vi "Teleop.vi"(10 "Match Info":T1={"Autonomous Elapsed Seconds"=0.0, "TeleOp Elapsed Seconds"=0.0, "Disabled Elapsed Seconds"=0.0, "Visited Autonomous"=FALSE, "Visited TeleOp"=FALSE, "Visited Disabled"=FALSE, "Autonomous Settings"={"Autonomous Style"=enum."Independent", "VI Refnum"=refnum}}, 11 "Call Context":T2) -> ()   [LabVIEW 2019]
doc: "This VI is called for each TeleOp packet received from the DS where the robot is not disabled. It is often used to read from the joysticks and update I/O or to update setpoints for timed control loops. It should complete and return within 20 milliseconds or it may miss DS packets."
uses:
  <vilib>/Rock Robotics/WPI/DriverStation/WPI_DriverStationDerivedRobotMode.ctl
  <vilib>/Rock Robotics/WPI/DriverStation/WPI_DriverStationMatch Info.ctl
  <vilib>/Rock Robotics/WPI/ThirdParty/Phoenix-LabVIEW/Motor Controller/Controls/CTRE_Phoenix_MotorControl_ControlMode.ctl
  <vilib>/Rock Robotics/WPI/Utilities/WPI_GetSetVariantRefNum.vi
  <vilib>/Rock Robotics/Network Tables/NT Write Boolean Array.vi
  <vilib>/Rock Robotics/Network Tables/NT Read Boolean.vi
  <vilib>/Rock Robotics/Network Tables/NT Read Number.vi
  <vilib>/Rock Robotics/Network Tables/NT Write Numeric Array.vi
panel:
  out "Sample Slider 0":dbl(slide) scale=0.0..5.0
  out "Sample Boolean 1":bool
  out "Sample Boolean 0":bool
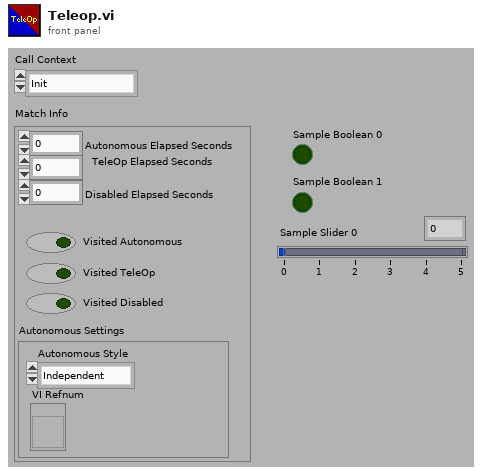
[diagram p1: front panel]
types:
  T1 = typedef "WPI_DriverStationMatch Info.ctl" = cluster{"Autonomous Elapsed Seconds":dbl, "TeleOp Elapsed Seconds":dbl, "Disabled Elapsed Seconds":dbl, "Visited Autonomous":bool, "Visited TeleOp":bool, "Visited Disabled":bool, "Autonomous Settings":cluster{"Autonomous Style":enum16{"Iterative", "Independent"}, "VI Refnum":refnum<vi>}}
  T2 = typedef "WPI_DriverStationDerivedRobotMode.ctl" = enum16{"Init", "Execute", "Stop"}
  T3 = typedef "WPI_JoystickDevRef.ctl" = cluster{"Device":T4}
  T4 = typedef "WPI_JoystickDeviceEnum.ctl" = enum16{"USB 0", "USB 1", "USB 2", "USB 3", "USB 4", "USB 5"}
  T5 = typedef "WPI_MotorControlDeviceRef.ctl" = cluster{"DeviceStatus":errorcluster, "Type":T6, "PWM":cluster{"PWM Channel":T7, "DeadBand":T8}, "CAN":cluster{"Device Number":u8, "SetOutput VI Ref":variant, "GetOutput VI Ref":variant, "Enable VI Ref":variant, "Disable VI Ref":variant, "Data":variant}, "Invert":bool, "DIO PWM":cluster{"PWM \"Enable\" Channel":T7, "DIOChannel":T9, "PWM Rate":dbl}}
  T6 = typedef "WPI_MotorControlType.ctl" = enum16{"PWM", "CAN", "DIO PWM"}
  T7 = typedef "FPGA_DIOPWMChannel.ctl" = enum8{"PWM 0", "PWM 1", "PWM 2", "PWM 3", "PWM 4", "PWM 5", "PWM 6", "PWM 7", "PWM 8", "PWM 9", "PWM MXP 0", "PWM MXP 1", "PWM MXP 2", "PWM MXP 3", "PWM MXP 4", "PWM MXP 5", "PWM MXP 6", "PWM MXP 7", "PWM MXP 8", "PWM MXP 9", "Invalid"}
  T8 = typedef "WPI_PWMDeadband.ctl" = cluster{"Name":string, "maxPositivePwm":i32, "minPositivePwm":i32, "centerPwm":i32, "maxNegativePwm":i32, "minNegativePwm":i32, "angularRange":u16}
  T9 = typedef "FPGA_DIOChannel.ctl" = enum8{"DIO 0", "DIO 1", "DIO 2", "DIO 3", "DIO 4", "DIO 5", "DIO 6", "DIO 7", "DIO 8", "DIO 9", "DIO MXP 0", "DIO MXP 1", "DIO MXP 2", "DIO MXP 3", "DIO MXP 4", "DIO MXP 5", "DIO MXP 6", "DIO MXP 7", "DIO MXP 8", "DIO MXP 9", "DIO MXP 10", "DIO MXP 11", "DIO MXP 12", "DIO MXP 13", "DIO MXP 14", "DIO MXP 15", "SPI Port CS1", "SPI Port CS2", "SPI Port CS3", "SPI Port MISO", "SPI Port MOSI", "Invalid"}
  T10 = typedef "CTRE_Phoenix_MotorControl_ControlMode.ctl" = u16
  T11 = typedef "WPI_RobotDriveDevRef.ctl" = cluster{"DevStatus":errorcluster, "Motors[]":T5[], "Square Inputs":bool, "Max Output":dbl}
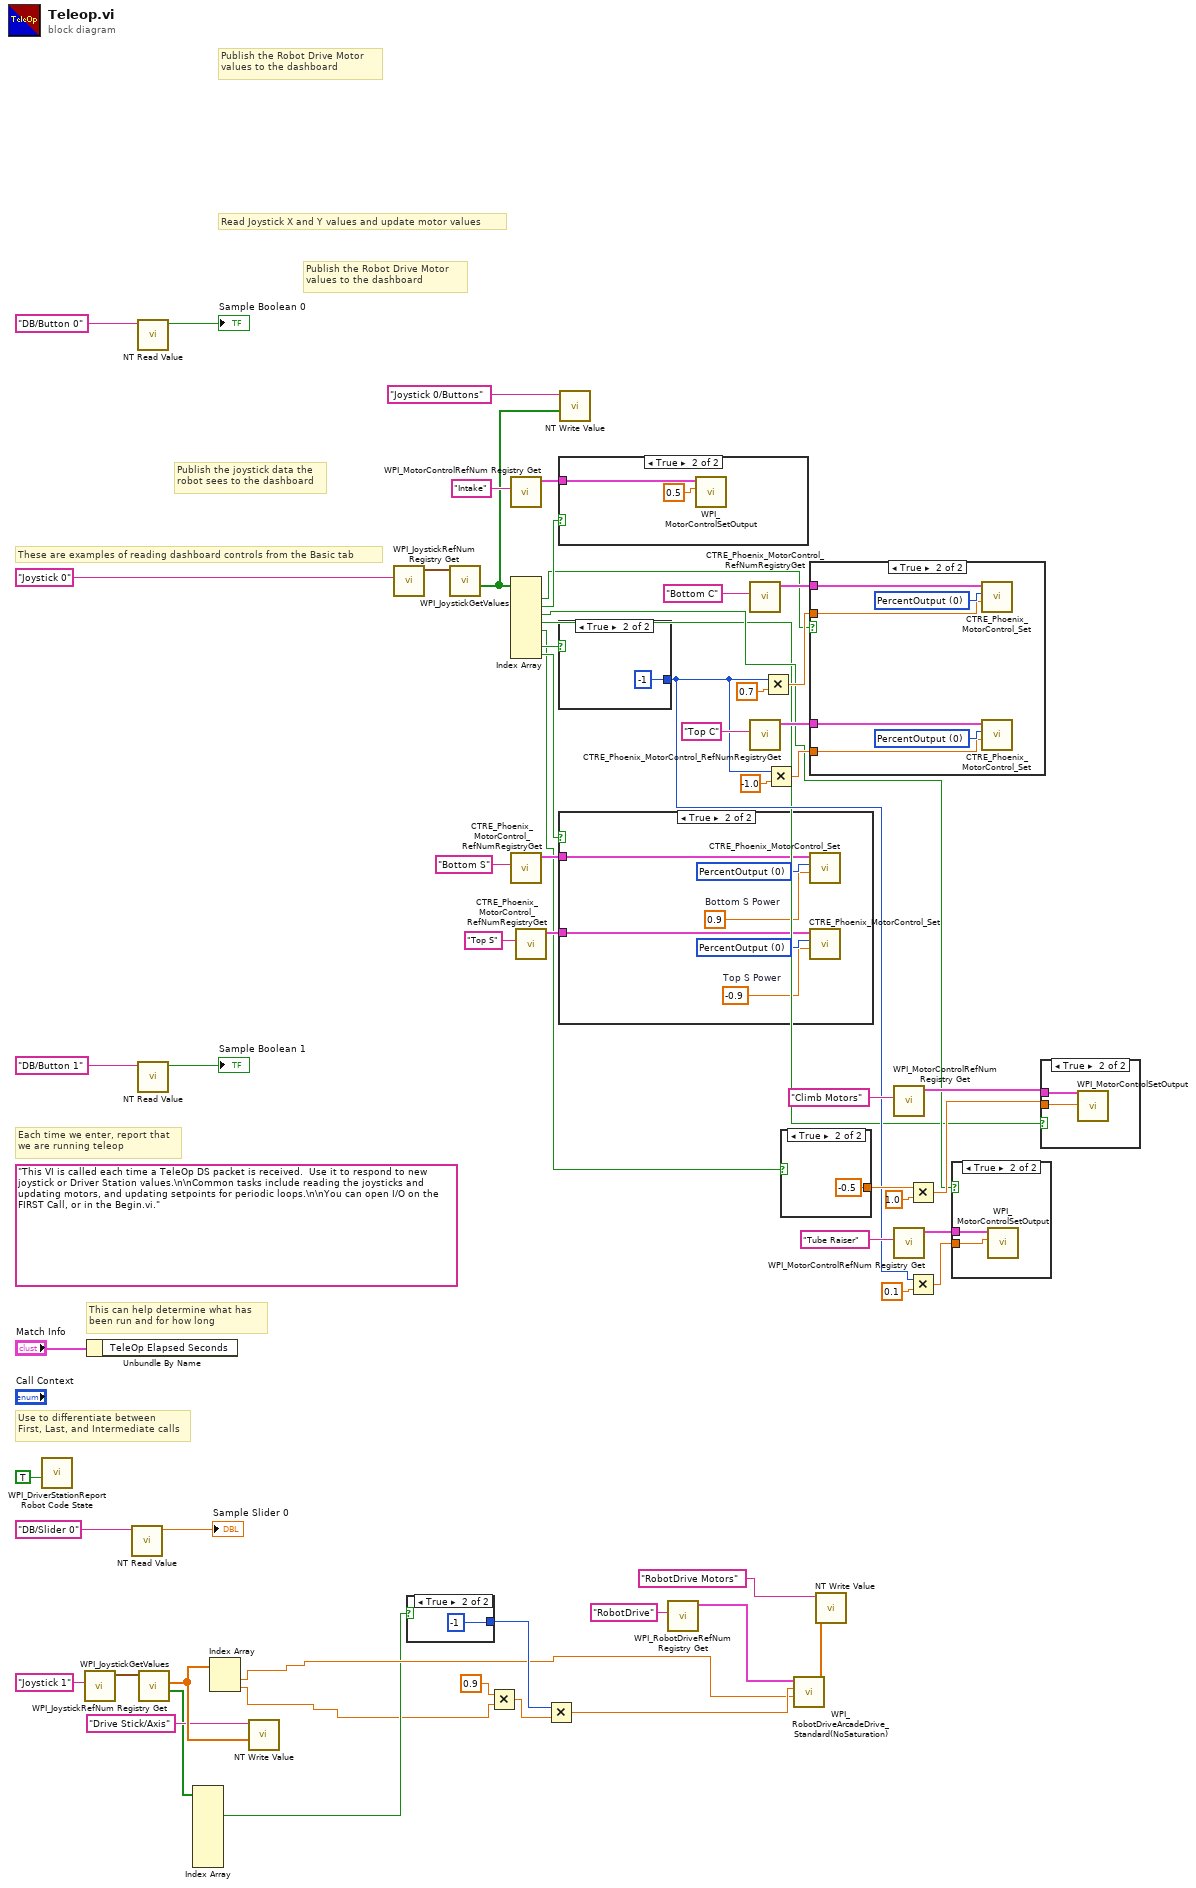
[diagram p0: block diagram]
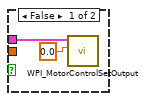
[diagram p2: hidden frame]
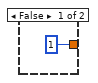
[diagram p3: hidden frame]
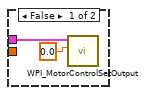
[diagram p4: hidden frame]
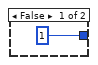
[diagram p5: hidden frame]
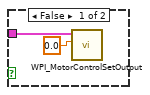
[diagram p6: hidden frame]
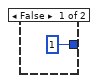
[diagram p7: hidden frame]
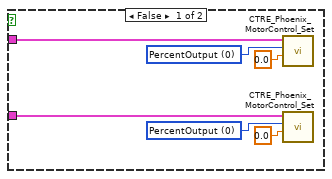
[diagram p8: hidden frame]
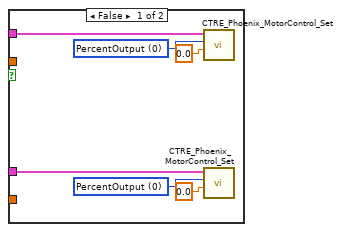
[diagram p9: hidden frame]
diagram:
  (unwired) "This VI is called each time a TeleOp DS packet is received.  Use it to respond to new joystick or Driver Station values.\n\nCommon tasks include reading the joysticks and updating motors, and updating setpoints for periodic loops.\n\nYou can open I/O on the FIRST Call, or in the Begin.vi."
  # "Publish the Robot Drive Motor\nvalues to the dashboard"
  # "These are examples of reading dashboard controls from the Basic tab"
  # "Publish the Robot Drive Motor\nvalues to the dashboard"
  # "Publish the joystick data the\nrobot sees to the dashboard"
  # "Each time we enter, report that\nwe are running teleop"
  # "Use to differentiate between\nFirst, Last, and Intermediate calls"
  # "This can help determine what has\nbeen run and for how long"
  # "Read Joystick X and Y values and update motor values"
  n1 = call <vilib>:"WPI_DriverStationReport Robot Code State.vi"("TeleOp"=TRUE ("Autonomous")) -> ()  [unwired: 10 in, 1 out]
  n2 = call <vilib>:"WPI_JoystickRefNum Registry Get.vi"("refnum name"="Joystick 1") -> ("JoystickDevRef"=w30:T3)  [unwired: 1 in, 9 out]
  n3 = Unbundle By Name("Match Info") -> ()  [unwired: 1 out]
  n4 = call-poly <vilib>:"NT Read Value.vi"("Name"="DB/Slider 0" ("refnum name")) -> ("Numeric"=→"Sample Slider 0":dbl)  [unwired: 9 in, 1 out]
  n5 = call-poly <vilib>:"NT Read Value.vi"("Name"="DB/Button 0" ("refnum name")) -> ("Boolean"=→"Sample Boolean 0":bool)  [unwired: 9 in, 1 out]
  n6 = call-poly <vilib>:"NT Read Value.vi"("Name"="DB/Button 1" ("refnum name")) -> ("Boolean"=→"Sample Boolean 1":bool)  [unwired: 9 in, 1 out]
  n7 = call <vilib>:"WPI_JoystickGetValues.vi"("JoystickDevRef"=w30) -> ("Buttons"=w23:bool[], "Axes"=w25:dbl[])  [unwired: 6 in, 3 out]
  n8 = Index Array(array=w23) -> (element #2=w5:bool)  [unwired: 8 in, 7 out]
  n9 = Index Array(array=w25) -> (element #1=w6:dbl, element #2=w3:dbl)  [unwired: 2 in]
  n10 = call-poly <vilib>:"NT Write Value.vi"("Numeric Array"=w25, "Name"="Drive Stick/Axis") -> ()  [unwired: 9 in, 1 out]
  n11 = call <vilib>:"WPI_JoystickRefNum Registry Get.vi"("refnum name"="Joystick 0") -> ("JoystickDevRef"=w57:T3)  [unwired: 1 in, 9 out]
  n12 = case shown="True" w5 {
    tunnel: [1 -1] -> w21
    frame False {
    }
    frame True {
    }
  }
  n13 = call <vilib>:"WPI_JoystickGetValues.vi"("JoystickDevRef"=w57) -> ("Buttons"=w34:bool[])  [unwired: 6 in, 4 out]
  n14 = Multiply(x=0.9, y=w3) -> (x*y=w2:dbl)
  n15 = call <vilib>:"WPI_MotorControlRefNum Registry Get.vi"("refnum name"="Intake") -> ("MotorControlDevRef"=w35:T5)  [unwired: 9 in, 1 out]
  n16 = Index Array(array=w34) -> (element #1=w1:bool, element #2=w32:bool, element #3=w8:bool, element #4=w7:bool, element #5=w9:bool, element #7=w22:bool, element #8=w33:bool)  [unwired: 8 in, 1 out]
  n17 = call <vilib>:"CTRE_Phoenix_MotorControl_RefNumRegistryGet.vi"("refnum name"="Bottom S") -> ("PhoenixMotorControlDevRef"=w44:T5)  [unwired: 9 in, 1 out]
  n18 = call <vilib>:"CTRE_Phoenix_MotorControl_RefNumRegistryGet.vi"("refnum name"="Top S") -> ("PhoenixMotorControlDevRef"=w41:T5)  [unwired: 9 in, 1 out]
  n19 = Multiply(x=w21, y=w2) -> (x*y=w20:dbl)
  n20 = case shown="True" w32 {
    tunnel: w35 -> [w62 w64]
    frame False {
      n21 = call <vilib>:"WPI_MotorControlSetOutput.vi"("Output"=0.0, "MotorControlDevRef"=w62) -> ()  [unwired: 7 in, 3 out]
    }
    frame True {
      n22 = call <vilib>:"WPI_MotorControlSetOutput.vi"("Output"=0.5, "MotorControlDevRef"=w64) -> ()  [unwired: 7 in, 3 out]
    }
  }
  n23 = case shown="True" w22 {
    tunnel: [1 -1] -> w10
    frame False {
    }
    frame True {
    }
  }
  n24 = case shown="True" w33 {
    tunnel: w44 -> [w71 w79]
    tunnel: w41 -> [w68 w76]
    frame False {
      w69 = T10 0 items=["PercentOutput"=0, "Position"=1, "Velocity"=2, "Current"=3, "Follower"=5, "MotionProfile"=6, "MotionMagic"=7, "MotionProfileArc"=10, "Disabled"=15] ("Control Mode")
      w72 = T10 0 items=["PercentOutput"=0, "Position"=1, "Velocity"=2, "Current"=3, "Follower"=5, "MotionProfile"=6, "MotionMagic"=7, "MotionProfileArc"=10, "Disabled"=15] ("Control Mode")
      n25 = call <vilib>:"CTRE_Phoenix_MotorControl_Set.vi"("Output"=0.0, "Control Mode"=w72, "PhoenixMotorControlDevRef"=w71) -> ()  [unwired: 7 in, 2 out]
      n26 = call <vilib>:"CTRE_Phoenix_MotorControl_Set.vi"("Output"=0.0, "Control Mode"=w69, "PhoenixMotorControlDevRef"=w68) -> ()  [unwired: 7 in, 2 out]
    }
    frame True {
      w74 = -0.9  # Top S Power
      w75 = 0.9  # Bottom S Power
      w77 = T10 0 items=["PercentOutput"=0, "Position"=1, "Velocity"=2, "Current"=3, "Follower"=5, "MotionProfile"=6, "MotionMagic"=7, "MotionProfileArc"=10, "Disabled"=15] ("Control Mode")
      w78 = T10 0 items=["PercentOutput"=0, "Position"=1, "Velocity"=2, "Current"=3, "Follower"=5, "MotionProfile"=6, "MotionMagic"=7, "MotionProfileArc"=10, "Disabled"=15] ("Control Mode")
      n27 = call <vilib>:"CTRE_Phoenix_MotorControl_Set.vi"("Output"=w75, "Control Mode"=w78, "PhoenixMotorControlDevRef"=w79) -> ()  [unwired: 7 in, 2 out]
      n28 = call <vilib>:"CTRE_Phoenix_MotorControl_Set.vi"("Output"=w74, "Control Mode"=w77, "PhoenixMotorControlDevRef"=w76) -> ()  [unwired: 7 in, 2 out]
    }
  }
  n29 = call-poly <vilib>:"NT Write Value.vi"("Boolean Array"=w34, "Name"="Joystick 0/Buttons") -> ()  [unwired: 9 in, 1 out]
  n30 = call <vilib>:"WPI_RobotDriveRefNum Registry Get.vi"("refnum name"="RobotDrive") -> ("RobotDriveDevRef"=w28:T11)  [unwired: 1 in, 9 out]
  n31 = call <vilib>:"CTRE_Phoenix_MotorControl_RefNumRegistryGet.vi"("refnum name"="Bottom C") -> ("PhoenixMotorControlDevRef"=w43:T5)  [unwired: 9 in, 1 out]
  n32 = call <vilib>:"CTRE_Phoenix_MotorControl_RefNumRegistryGet.vi"("refnum name"="Top C") -> ("PhoenixMotorControlDevRef"=w47:T5)  [unwired: 9 in, 1 out]
  n33 = Multiply(x=w10, y=0.7 ("Output")) -> (x*y=w37:dbl)
  n34 = Multiply(x=w10, y=-1.0 ("Output")) -> (x*y=w39:dbl)
  n35 = case shown="True" w9 {
    tunnel: [1 -0.5] -> w11
    frame False {
    }
    frame True {
    }
  }
  n36 = call <vilib>:"WPI_RobotDriveArcadeDrive_Standard(NoSaturation).vi"("Y axis value"=w6, "X axis value"=w20, "RobotDriveDevRef"=w28) -> ("Motor Values"=w27:dbl[])  [unwired: 1 in, 7 out]
  n37 = case shown="True" w1 {
    tunnel: w47 -> [w85 w93]
    tunnel: w43 -> [w82 w90]
    tunnel: w39 -> [_ w89]
    tunnel: w37 -> [_ w88]
    frame False {
      w83 = T10 0 items=["PercentOutput"=0, "Position"=1, "Velocity"=2, "Current"=3, "Follower"=5, "MotionProfile"=6, "MotionMagic"=7, "MotionProfileArc"=10, "Disabled"=15] ("Control Mode")
      w86 = T10 0 items=["PercentOutput"=0, "Position"=1, "Velocity"=2, "Current"=3, "Follower"=5, "MotionProfile"=6, "MotionMagic"=7, "MotionProfileArc"=10, "Disabled"=15] ("Control Mode")
      n38 = call <vilib>:"CTRE_Phoenix_MotorControl_Set.vi"("Output"=0.0, "Control Mode"=w83, "PhoenixMotorControlDevRef"=w82) -> ()  [unwired: 7 in, 2 out]
      n39 = call <vilib>:"CTRE_Phoenix_MotorControl_Set.vi"("Output"=0.0, "Control Mode"=w86, "PhoenixMotorControlDevRef"=w85) -> ()  [unwired: 7 in, 2 out]
    }
    frame True {
      w91 = T10 0 items=["PercentOutput"=0, "Position"=1, "Velocity"=2, "Current"=3, "Follower"=5, "MotionProfile"=6, "MotionMagic"=7, "MotionProfileArc"=10, "Disabled"=15] ("Control Mode")
      w92 = T10 0 items=["PercentOutput"=0, "Position"=1, "Velocity"=2, "Current"=3, "Follower"=5, "MotionProfile"=6, "MotionMagic"=7, "MotionProfileArc"=10, "Disabled"=15] ("Control Mode")
      n40 = call <vilib>:"CTRE_Phoenix_MotorControl_Set.vi"("Output"=w88, "Control Mode"=w91, "PhoenixMotorControlDevRef"=w90) -> ()  [unwired: 7 in, 2 out]
      n41 = call <vilib>:"CTRE_Phoenix_MotorControl_Set.vi"("Output"=w89, "Control Mode"=w92, "PhoenixMotorControlDevRef"=w93) -> ()  [unwired: 7 in, 2 out]
    }
  }
  n42 = call-poly <vilib>:"NT Write Value.vi"("Numeric Array"=w27, "Name"="RobotDrive Motors") -> ()  [unwired: 9 in, 1 out]
  n43 = call <vilib>:"WPI_MotorControlRefNum Registry Get.vi"("refnum name"="Climb Motors") -> ("MotorControlDevRef"=w14:T5)  [unwired: 9 in, 1 out]
  n44 = call <vilib>:"WPI_MotorControlRefNum Registry Get.vi"("refnum name"="Tube Raiser") -> ("MotorControlDevRef"=w18:T5)  [unwired: 9 in, 1 out]
  n45 = Multiply(x=w11, y=1.0 ("Output")) -> (x*y=w12:dbl)
  n46 = Multiply(x=w10, y=0.1 ("Output")) -> (x*y=w16:dbl)
  n47 = case shown="True" w8 {
    tunnel: w18 -> [w94 w97]
    tunnel: w16 -> [_ w96]
    frame False {
      n48 = call <vilib>:"WPI_MotorControlSetOutput.vi"("Output"=0.0, "MotorControlDevRef"=w94) -> ()  [unwired: 7 in, 3 out]
    }
    frame True {
      n49 = call <vilib>:"WPI_MotorControlSetOutput.vi"("Output"=w96, "MotorControlDevRef"=w97) -> ()  [unwired: 7 in, 3 out]
    }
  }
  n50 = case shown="True" w7 {
    tunnel: w14 -> [w98 w101]
    tunnel: w12 -> [_ w100]
    frame False {
      n51 = call <vilib>:"WPI_MotorControlSetOutput.vi"("Output"=0.0, "MotorControlDevRef"=w98) -> ()  [unwired: 7 in, 3 out]
    }
    frame True {
      n52 = call <vilib>:"WPI_MotorControlSetOutput.vi"("Output"=w100, "MotorControlDevRef"=w101) -> ()  [unwired: 7 in, 3 out]
    }
  }
